vi "NXT Relay Driver.vi"(0 "Relay":u16(ring) items=["Off", "Relay 1", "Relay 2"], 2 "NXT":T2={"Hardware"="NXT", "Flattened String"=""}, 3 "Input Port":T1 items=["Port 1", "Port 2", "Port 3", "Port 4"]) -> (4 "NXT dup":T2={"Hardware"="NXT", "Flattened String"=""} caption="NXT")   [LabVIEW 2010]
uses:
  <vilib>/NXT/Subs/LVHSConnector.ctl
  <vilib>/NXT/Block Support/NXT_InputPort.ctl
  <vilib>/NXT/Block Support/HWPage.SensorType.ctl
  <vilib>/NXT/Block Support/HWPage.SensorMode.ctl
  <vilib>/NXT/Dual Mode Library/Motors/MotorBrake.vi
  <vilib>/NXT/Dual Mode Library/Motors/MotorOn.vi
  <vilib>/NXT/Dual Mode Library/Motors/MotorReverse.vi
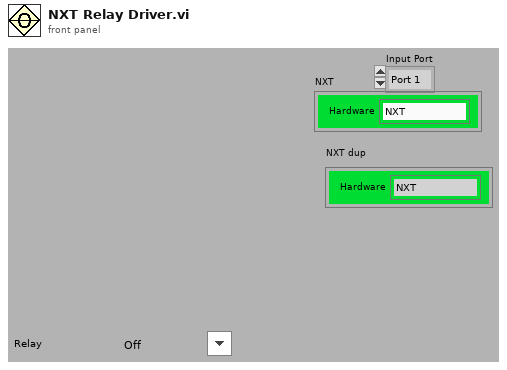
[diagram p1: front panel]
types:
  T1 = typedef "NXT_InputPort.ctl" = u8
  T2 = typedef "LVHSConnector.ctl" = cluster{"Hardware":string, "Flattened String":string}
  T3 = typedef "HWPage.SensorType.ctl" = u8
  T4 = typedef "HWPage.SensorMode.ctl" = u8
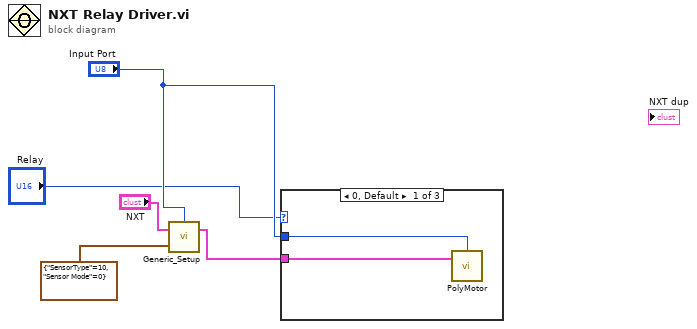
[diagram p0: block diagram]
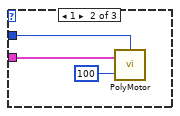
[diagram p2: hidden frame]
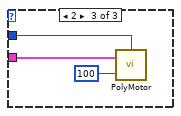
[diagram p3: hidden frame]
diagram:
  n1 = call <vilib>:"Generic_Setup.vi"("Sensor Setup"=cluster{"SensorType":T3, "Sensor Mode":T4} {"SensorType"=10, "Sensor Mode"=0}, "NXT"="NXT", "Port"="Input Port") -> ("NXT"=w2:T2)  [unwired: 1 out]
  n2 = case shown="0, Default" "Relay" {
    tunnel: w2 -> [w7 w9 w13]
    tunnel: "Input Port" -> [w6 w8 w11]
    frame 0, Default {
      n3 = call-poly <vilib>:"PolyMotor.vi"("NXT"=w7, "Port (All Ports)"=w6) -> ()  [unwired: 2 in, 1 out]
    }
    frame 1 {
      n4 = call-poly <vilib>:"PolyMotor.vi"("Power (75)"=100, "NXT"=w9, "Output Port (All Ports)"=w8) -> ()  [unwired: 1 in, 1 out]
    }
    frame 2 {
      n5 = call-poly <vilib>:"PolyMotor.vi"("Power (75)"=100, "NXT"=w13, "Output Port (All Ports)"=w11) -> ()  [unwired: 1 in, 1 out]
    }
  }
